vi "Associated Power Technologies 8500 Series Pulse Mode.vi"() -> ()   [LabVIEW 2014]
doc: "This VI is an example for controlling the power source, APT-8500 series, of Associated Power Technologies. \n\nThis VI shows how to configure the pulse mode and output."
uses:
  <instrlib>/Associated Power Technologies 8500 Series/Public/Configure/Pulse Mode/Pulse Mode - Add File.vi
  <instrlib>/Associated Power Technologies 8500 Series/Public/Configure/Pulse Mode/Pulse Mode - Edit File.vi
  <instrlib>/Associated Power Technologies 8500 Series/Public/Configure/Pulse Mode/Pulse Mode - Configure File Loop.vi
  <instrlib>/Associated Power Technologies 8500 Series/Public/Configure/Pulse Mode/Pulse Mode - Configure Trigger Source.vi
  <instrlib>/Associated Power Technologies 8500 Series/Public/Configure/Pulse Mode/Pulse Mode - Configure Range.vi
  <instrlib>/Associated Power Technologies 8500 Series/Public/Configure/Pulse Mode/Pulse Mode - Configure AC Voltage.vi
  <instrlib>/Associated Power Technologies 8500 Series/Public/Configure/Pulse Mode/Pulse Mode - Configure Frequency.vi
  <instrlib>/Associated Power Technologies 8500 Series/Public/Configure/Pulse Mode/Pulse Mode - Configure DC Voltage.vi
  <instrlib>/Associated Power Technologies 8500 Series/Public/Configure/Pulse Mode/Pulse Mode - Configure Start Angle.vi
  <instrlib>/Associated Power Technologies 8500 Series/Public/Configure/Pulse Mode/Pulse Mode - Configure Transient AC Voltage.vi
  <instrlib>/Associated Power Technologies 8500 Series/Public/Configure/Pulse Mode/Pulse Mode - Configure Transient DC Voltage.vi
  <instrlib>/Associated Power Technologies 8500 Series/Public/Configure/Pulse Mode/Pulse Mode - Configure Duty Cycle.vi
  <instrlib>/Associated Power Technologies 8500 Series/Public/Configure/Pulse Mode/Pulse Mode - Configure Period.vi
  <instrlib>/Associated Power Technologies 8500 Series/Public/Configure/Pulse Mode/Pulse Mode - Load File.vi
  <instrlib>/Associated Power Technologies 8500 Series/Public/Data/Measurement/Read All Measurements.vi
  <instrlib>/Associated Power Technologies 8500 Series/Associated Power Technologies 8500 Series.lvlib
panel:
  out "All Measurements":T1
  in  "Pulse Mode Configurations":T2={"Loop Count"=800, "Trigger Source"=0, "Range"=0, "AC Voltage"=20.0, "Frequency"=50.0, "DC Voltage"=0.0, "Start Angle(degree)"=0, "Transient AC Voltage"=20.0, "Transient DC Voltage"=0.0, "Duty Cycle (0-100)"=50, "Period"=10.0} {"Loop Count" max=5000; "Trigger Source" items=["AUTO", "MANUAL"]; "Range" items=["AUTO", "HIGH", "LOW"]; "AC Voltage" min=0.0 max=310.0; "Frequency" min=5.0 max=1200.0; "DC Voltage" min=0.0 max=420.0; "Start Angle(degree)" max=359; "Transient AC Voltage" min=0.0 max=310.0; "Transient DC Voltage" min=0.0 max=420.0; "Duty Cycle (0-100)" max=100; "Period" min=0.1 max=999.9 step=0.1}
  in  "Stop":bool
  in  "Serial Configuration":T3={"Baud Rate"=115200, "Parity"=0, "Data Bits"=8, "Stop Bits"=10, "Flow Control"=0} {"Flow Control" items=["None", "XON/XOFF", "RTS/CTS", "XON/XOFF & RTS/CTS", "DTR/DSR", "XON/XOFF & DTR/DSR"]; "Stop Bits" items=["1.0"=10, "1.5"=15, "2.0"=20]; "Data Bits" items=["7"=7, "8"=8]; "Parity" items=["None", "Odd", "Even", "Mark", "Space"]; "Baud Rate" items=["300"=300, "600"=600, "1200"=1200, "2400"=2400, "4800"=4800, "9600"=9600, "19200"=19200, "38400"=38400, "115200"=115200]}
  in  "VISA resource name":refnum<visa-resource-name>
  # "Pulse Mode Operation of APT-8500 Series"
  # "Initialization"
  # "Configurations"
  # "Meters"
  # "(c) 2020 Associated Power Technologies.  ALL RIGHTS RESERVED."
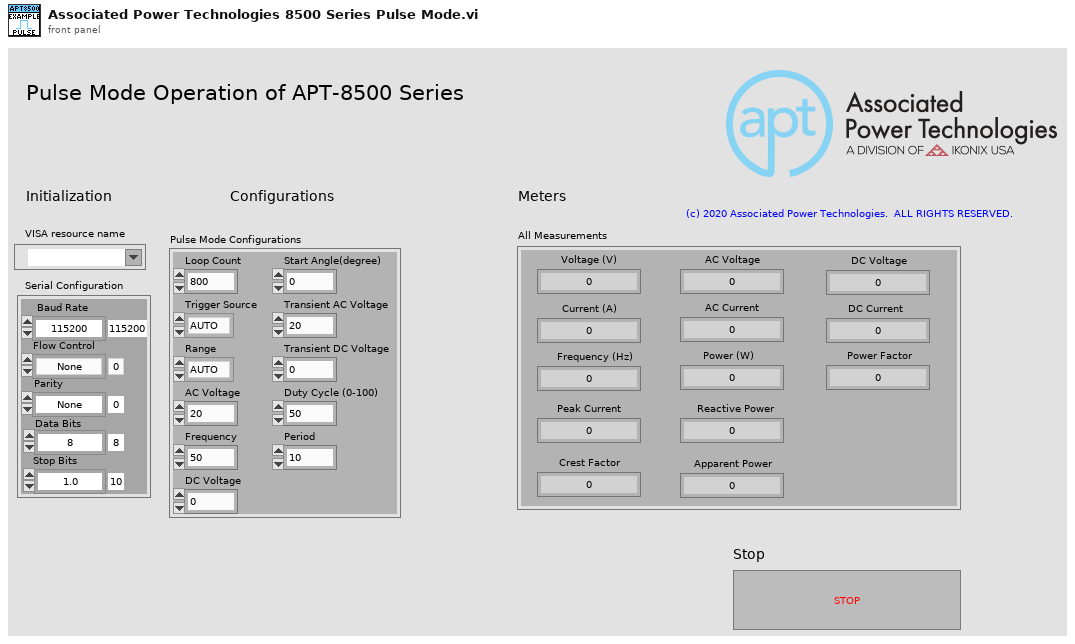
[diagram p1: front panel]
types:
  T1 = cluster{"Voltage (V)":dbl, "AC Voltage":dbl, "DC Voltage":dbl, "Current (A)":dbl, "AC Current":dbl, "DC Current":dbl, "Frequency (Hz)":dbl, "Power (W)":dbl, "Power Factor":dbl, "Peak Current":dbl, "Reactive Power":dbl, "Crest Factor":dbl, "Apparent Power":dbl}
  T2 = cluster{"Loop Count":u16, "Trigger Source":u16, "Range":u16, "AC Voltage":dbl, "Frequency":dbl, "DC Voltage":dbl, "Start Angle(degree)":u16, "Transient AC Voltage":dbl, "Transient DC Voltage":dbl, "Duty Cycle (0-100)":u16, "Period":dbl}
  T3 = cluster{"Baud Rate":u32, "Parity":u16, "Data Bits":u16, "Stop Bits":u16, "Flow Control":u16}
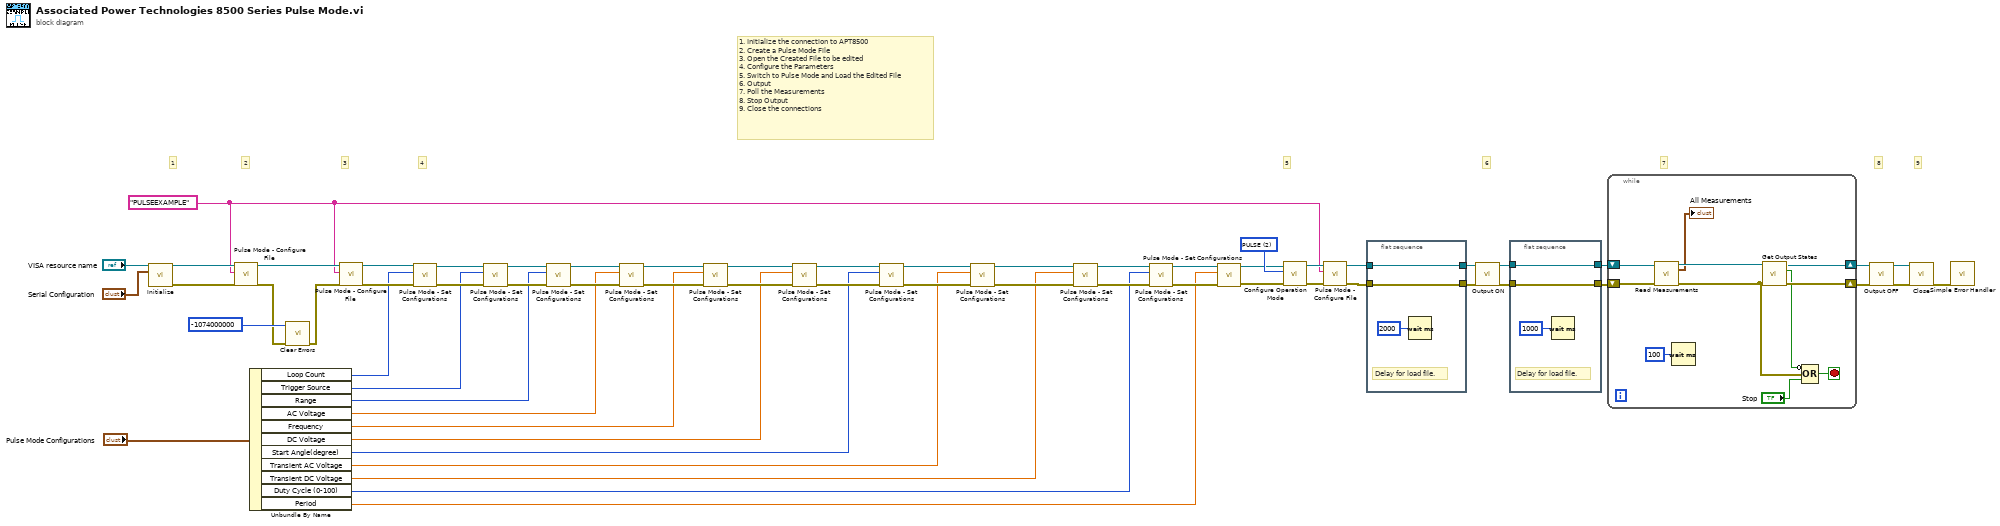
[diagram p0: block diagram]
diagram:
  w41 = "PULSEEXAMPLE" ("File Name")
  w42 = u16 2 items=["MANUAL", "LIST", "PULSE", "STEP"] ("Operation Mode")
  # "1. Initialize the connection to APT8500\n2. Create a Pulse Mode File\n3. Open the Created File to be edited\n4. Configure the Parameters\n5. Switch to Pulse Mode and Load the Edited File\n6. Output\n7. Poll the Measurements\n8. Stop Output\n9. Close the connections"
  # "9"
  # "8"
  # "7"
  # "6"
  # "5"
  # "4"
  # "3"
  # "2"
  # "1"
  n1 = call <instrlib>:"Initialize.vi"("VISA resource name"="VISA resource name", "Serial Configuration"="Serial Configuration") -> ("VISA resource name out"=w61:refnum<visa-resource-name>, "error out"=w60:errorcluster)  [unwired: 12 in]
  n2 = call-poly <instrlib>:"Pulse Mode - Configure File.vi"("error in (no error)"=w60, "File Name"=w41, "VISA resource name"=w61) -> ("error out"=w55:errorcluster, "VISA resource name out"=w57:refnum<visa-resource-name>)  [unwired: 7 in]
  n3 = Unbundle By Name("Pulse Mode Configurations") -> ("Loop Count"=w13:u16, "Trigger Source"=w12:u16, "Range"=w11:u16, "AC Voltage"=w10:dbl, "Frequency"=w9:dbl, "DC Voltage"=w8:dbl, "Start Angle(degree)"=w7:u16, "Transient AC Voltage"=w6:dbl, "Transient DC Voltage"=w5:dbl, "Duty Cycle (0-100)"=w4:u16, "Period"=w3:dbl)
  n4 = call <vilib>:"Clear Errors.vi"("error in (no error)"=w55, "specific error code to clear (0: all)"=-1074000000) -> ("error out"=w54:errorcluster)  [unwired: 4 in, 1 out]
  n5 = call-poly <instrlib>:"Pulse Mode - Configure File.vi"("error in (no error)"=w54, "File Name"=w41, "VISA resource name"=w57) -> ("error out"=w35:errorcluster, "VISA resource name out"=w36:refnum<visa-resource-name>)  [unwired: 7 in]
  n6 = call-poly <instrlib>:"Pulse Mode - Set Configurations.vi"("error in (no error)"=w35, "Loop Count (0)"=w13, "VISA resource name"=w36) -> ("error out"=w33:errorcluster, "VISA resource name out"=w34:refnum<visa-resource-name>)  [unwired: 7 in]
  n7 = call-poly <instrlib>:"Pulse Mode - Set Configurations.vi"("error in (no error)"=w33, "Trigger Source"=w12, "VISA resource name"=w34) -> ("error out"=w31:errorcluster, "VISA resource name out"=w32:refnum<visa-resource-name>)  [unwired: 7 in]
  n8 = call-poly <instrlib>:"Pulse Mode - Set Configurations.vi"("error in (no error)"=w31, "Range"=w11, "VISA resource name"=w32) -> ("error out"=w29:errorcluster, "VISA resource name out"=w30:refnum<visa-resource-name>)  [unwired: 7 in]
  n9 = call-poly <instrlib>:"Pulse Mode - Set Configurations.vi"("error in (no error)"=w29, "AC Voltage"=w10, "VISA resource name"=w30) -> ("error out"=w27:errorcluster, "VISA resource name out"=w28:refnum<visa-resource-name>)  [unwired: 7 in]
  n10 = call-poly <instrlib>:"Pulse Mode - Set Configurations.vi"("error in (no error)"=w27, "Frequency (60)"=w9, "VISA resource name"=w28) -> ("error out"=w25:errorcluster, "VISA resource name out"=w26:refnum<visa-resource-name>)  [unwired: 7 in]
  n11 = call-poly <instrlib>:"Pulse Mode - Set Configurations.vi"("error in (no error)"=w25, "DC Voltage"=w8, "VISA resource name"=w26) -> ("error out"=w23:errorcluster, "VISA resource name out"=w24:refnum<visa-resource-name>)  [unwired: 7 in]
  n12 = call-poly <instrlib>:"Pulse Mode - Set Configurations.vi"("error in (no error)"=w23, "Start Angle(degree)"=w7, "VISA resource name"=w24) -> ("error out"=w22:errorcluster, "VISA resource name out"=w21:refnum<visa-resource-name>)  [unwired: 7 in]
  n13 = call-poly <instrlib>:"Pulse Mode - Set Configurations.vi"("error in (no error)"=w22, "Transient AC Voltage"=w6, "VISA resource name"=w21) -> ("error out"=w19:errorcluster, "VISA resource name out"=w20:refnum<visa-resource-name>)  [unwired: 7 in]
  n14 = call-poly <instrlib>:"Pulse Mode - Set Configurations.vi"("error in (no error)"=w19, "Transient DC Voltage"=w5, "VISA resource name"=w20) -> ("error out"=w17:errorcluster, "VISA resource name out"=w18:refnum<visa-resource-name>)  [unwired: 7 in]
  n15 = call-poly <instrlib>:"Pulse Mode - Set Configurations.vi"("error in (no error)"=w17, "Duty Cycle (0)"=w4, "VISA resource name"=w18) -> ("error out"=w15:errorcluster, "VISA resource name out"=w16:refnum<visa-resource-name>)  [unwired: 7 in]
  n16 = call-poly <instrlib>:"Pulse Mode - Set Configurations.vi"("error in (no error)"=w15, "Period (0.2)"=w3, "VISA resource name"=w16) -> ("error out"=w1:errorcluster, "VISA resource name out"=w2:refnum<visa-resource-name>)  [unwired: 7 in]
  n17 = call <instrlib>:"Configure Operation Mode.vi"("error in (no error)"=w1, "Operation Mode (MANUAL)"=w42, "VISA resource name"=w2) -> ("error out"=w43:errorcluster, "VISA resource name out"=w44:refnum<visa-resource-name>)  [unwired: 7 in]
  n18 = call-poly <instrlib>:"Pulse Mode - Configure File.vi"("error in (no error)"=w43, "File Name"=w41, "VISA resource name"=w44) -> ("error out"=w46:errorcluster, "VISA resource name out"=w48:refnum<visa-resource-name>)  [unwired: 7 in]
  n19 = flat-sequence {
    tunnel: [w64] -> w49
    tunnel: w48 -> [w64]
    tunnel: [w63] -> w47
    tunnel: w46 -> [w63]
    frame #0 {
      # "Delay for load file."
      n20 = Wait (ms)(milliseconds to wait=u32 2000) -> ()  [unwired: 1 out]
    }
  }
  n21 = call <instrlib>:"Output ON.vi"("VISA resource name"=w49, "error in (no error)"=w47) -> ("VISA resource name out"=w37:refnum<visa-resource-name>, "error out"=w39:errorcluster)  [unwired: 12 in]
  n22 = flat-sequence {
    tunnel: [w66] -> w40
    tunnel: w39 -> [w66]
    tunnel: [w65] -> w38
    tunnel: w37 -> [w65]
    frame #0 {
      # "Delay for load file."
      n23 = Wait (ms)(milliseconds to wait=u32 1000) -> ()  [unwired: 1 out]
    }
  }
  n24 = while {
    shift-right: [w72] -> w52
    shift-left: w38 -> [w76]
    shift-right: [w70] -> w53
    shift-left: w40 -> [w75]
    stop <- w78 stop-if-true
    n25 = call-poly <instrlib>:"Read Measurements.vi"("VISA resource name"=w76, "error in (no error)"=w75) -> ("VISA resource name out"=w73:refnum<visa-resource-name>, "All Measurements"=→"All Measurements":T1, "error out"=w71:errorcluster)  [unwired: 11 in]
    n26 = Wait (ms)(milliseconds to wait=u32 100) -> ()  [unwired: 1 out]
    n27 = call <instrlib>:"Get Output States.vi"("error in (no error)"=w71, "VISA resource name"=w73) -> ("error out"=w70:errorcluster, "Output?"=w69:bool, "VISA resource name out"=w72:refnum<visa-resource-name>)  [unwired: 7 in]
    n28 = Compound Arithmetic op=OR(invert w69, w71, "Stop") -> (w78:bool)
  }
  n29 = call <instrlib>:"Output OFF.vi"("VISA resource name"=w52, "error in (no error)"=w53) -> ("VISA resource name out"=w51:refnum<visa-resource-name>, "error out"=w50:errorcluster)  [unwired: 12 in]
  n30 = call <instrlib>:"Close.vi"("VISA resource name"=w51, "error in (no error)"=w50) -> ("error out"=w45:errorcluster)  [unwired: 13 in]
  n31 = call <vilib>:"Simple Error Handler.vi"("error in (no error)"=w45) -> ()  [unwired: 4 in, 5 out]
